vi "Connect.vi"(8 "error in":errorcluster, 11 "EF20 in":refnum<class "EF20.lvclass">) -> (0 "error out":errorcluster, 3 "EF20 out":refnum<class "EF20.lvclass">)   [LabVIEW 2018, in "EF20.lvlib" / "EF20.lvclass"]
uses:
  EF20.lvclass
  <vilib>/Instr/_visa.llb/VISA Configure Serial Port (Instr).vi
  PPLs/Oven/Oven.lvlibp/Oven.lvclass
  C:/Projects/LabVIEW/PPLs/Oven/Oven.lvlibp/Oven.lvclass
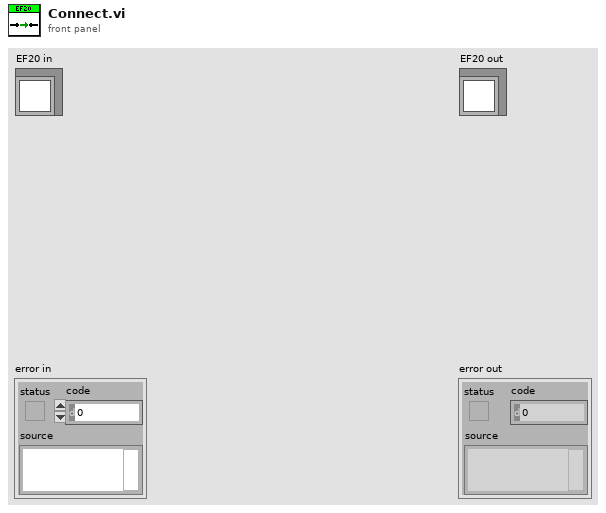
[diagram p1: front panel]
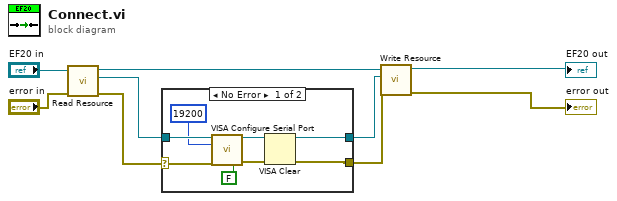
[diagram p0: block diagram]
diagram:
  n1 = call "Read Resource.vi"("error in (no error)"="error in", "Oven in"="EF20 in") -> ("error out"=w4:errorcluster, "Resource"=w3:refnum<visa-resource-name>, "Oven out"=w5:refnum<class "EF20.lvclass">)  [unwired: 7 in]
  n2 = case shown="No Error" w4 {
    selector: w4 -> [w14 w18]
    tunnel: w3 -> [w17 w19]
    tunnel: [w13 w19] -> w2
    tunnel: [w11 w18] -> w1
    frame No Error {
      n3 = call-poly "VISA Configure Serial Port"("VISA resource name"=w17, "Enable Termination\nChar (T)"=FALSE ("Enable Termination\nChar (T)"), "baud rate (9600)"=u32 19200, "error in (no error)"=w14) -> ("VISA resource name out"=w15:refnum<visa-resource-name>, "error out"=w12:errorcluster)  [unwired: 10 in]
      n4 = VISA Clear(VISA resource name=w15, error in (no error)=w12) -> (VISA resource name out=w13:refnum<visa-resource-name>, error out=w11:errorcluster)
    }
    frame Error {
    }
  }
  n5 = call "Write Resource.vi"("error in (no error)"=w1, "Resource"=w2, "Oven in"=w5) -> ("error out"=→"error out":errorcluster, "Oven out"=→"EF20 out":refnum<class "EF20.lvclass">)  [unwired: 7 in]
